vi "CoriFlowBFS1Plus_Init.vi"(0 "object in":refnum<class "CoriFlowBFS1Plus.lvclass">, 2 "VISA resource name":refnum<visa-resource-name>, 3 "Filter(0-1)Min-Max":dbl min=0.0 max=1.0, 4 "SW Buffer Size":i32, 5 "error in (no error)":errorcluster, 8 "Sample Rate (Hz)":dbl=10.0) -> (14 "object out":refnum<class "CoriFlowBFS1Plus.lvclass">, 19 "error out":errorcluster)   [LabVIEW 2023, in "CoriFlowBFS1Plus.lvclass"]
uses:
  CoriFlowBFS1Plus.lvclass
  CoriFlowBFS1Plus.lvclass/CoriFlowBFS1Plus.ctl
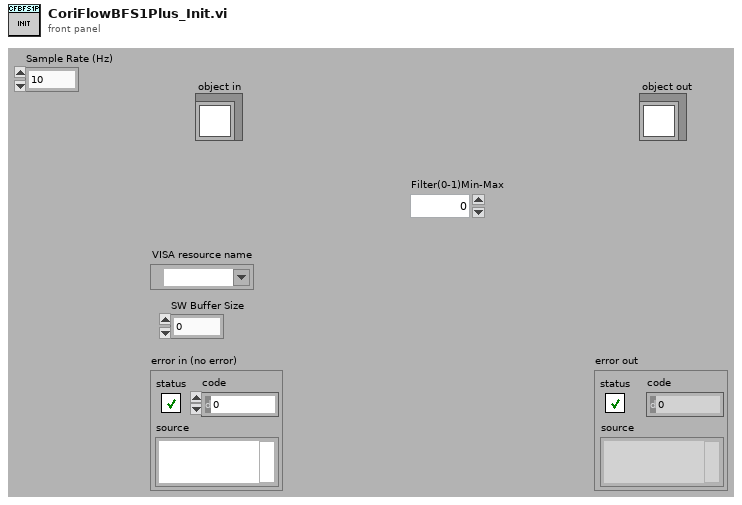
[diagram p1: front panel]
types:
  T1 = enum32{"Invalid", "Standard", "Closed", "Hidden", "Minimized", "Maximized"}
  T2 = cluster{"Message":string, "Message Data":variant}
  T3 = cluster{"Cluster":cluster{"Density_g_L":sgl, "FLow(ul/min)":sgl, "Temperature(C)":sgl}, "current time":timestamp}
  T4 = typedef "Z_BFS_type.ctl" = cluster{"VISA_Name":refnum<visa-resource-name>, "density_g_L":dbl, "Capacity":dbl, "Capacity units conversion":dbl}
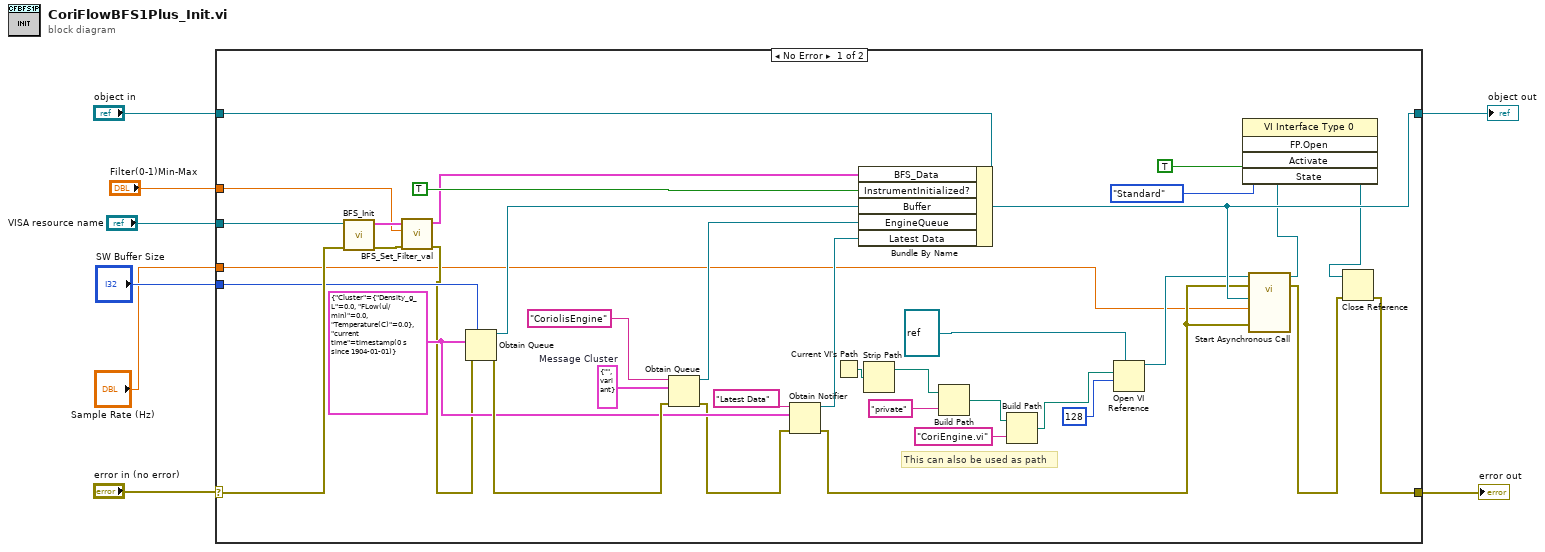
[diagram p0: block diagram]
diagram:
  n1 = case shown="No Error" "error in (no error)" {
    selector: "error in (no error)" -> [w43 w46]
    tunnel: "object in" -> [w45 w47]
    tunnel: [w20 w47] -> w7
    tunnel: [w16 w46] -> w5
    tunnel: "VISA resource name" -> [w44 _]
    tunnel: "Filter(0-1)Min-Max" -> [w39 _]
    tunnel: "SW Buffer Size" -> [w38 _]
    tunnel: "Sample Rate (Hz)" -> [w13 _]
    frame No Error {
      w36 = T2 {"Message"="", "Message Data"=variant}  # Message Cluster
      w32 = T3 {"Cluster"={"Density_g_L"=0.0, "FLow(ul/min)"=0.0, "Temperature(C)"=0.0}, "current time"=timestamp(0 s since 1904-01-01)}
      # "This can also be used as path"
      n2 = call "BFS_Init.vi"("error in"=w43, "VISA resource name"=w44) -> ("error out"=w28:errorcluster, "BFS_Out"=w41:T4)  [unwired: 8 in]
      n3 = call "BFS_Set_Filter_val.vi"("error in (no error)"=w28, "Sensor_Filter_0_to_1"=w39, "BFS_type_In"=w41) -> ("error out"=w27:errorcluster, "BFS_type_Out"=w40:T4)  [unwired: 7 in]
      n4 = Obtain Queue(max queue size (-1, unlimited)=w38, element data type=w32, error in (no error)=w27) -> (queue out=w37:refnum<queue>, error out=w35:errorcluster)  [unwired: 2 in, 1 out]
      n5 = Obtain Queue(name (unnamed)="CoriolisEngine", element data type=w36, error in (no error)=w35) -> (queue out=w33:refnum<queue>, error out=w30:errorcluster)  [unwired: 2 in, 1 out]
      n6 = Obtain Notifier(name (unnamed)="Latest Data", notification data type=w32, error in (no error)=w30) -> (notifier out=w29:refnum<notifier>, error out=w19:errorcluster)  [unwired: 1 in, 1 out]
      n7 = Current VI's Path() -> (path=w24:path)
      n8 = Bundle By Name(cluster=w45, "BFS_Data"=w40, "InstrumentInitialized?"=TRUE, "Buffer"=w37, "EngineQueue"=w33, "Latest Data"=w29) -> (w20:refnum<class "CoriFlowBFS1Plus.lvclass">)
      n9 = Strip Path(path=w24) -> (stripped path=w25:path)  [unwired: 1 out]
      n10 = Build Path(base path=w25, name or relative path="private") -> (appended path=w26:path)
      n11 = Build Path(base path=w26, name or relative path="CoriEngine.vi") -> (appended path=w14:path)
      n12 = Open VI Reference(type specifier VI Refnum (for type only)=refnum<vi> refnum, vi path=w14, options=128) -> (vi reference=w18:refnum<vi>)  [unwired: 3 in, 1 out]
      n13 = call-by-ref "Start Asynchronous Call"(reference=w18, error in=w19, "object in"=w20, "Sample Rate (Hz)"=w13, 5:"error in (no error)"=w19) -> (reference out=w10:refnum<vi>, error out=w17:errorcluster)  [unwired: 15 in, 2 out]
      n14 = invoke class="VI Interface Type 0" method="FP.Open"(reference=w10, "Activate"=TRUE ("Activate?"), "State"=T1."Standard") -> (reference out=w9:refnum<vi>)  [unwired: 2 in, 4 out]
      n15 = Close Reference(reference=w9, error in (no error)=w17) -> (error out=w16:errorcluster)
    }
    frame Error {
    }
  }
  "object out" <- w7
  "error out" <- w5
